vi "Periodic Tasks.vi"   [LabVIEW 2016]
doc: "This VI runs in parallel to other tasks. It can contain as many user-defined periodic loops as you need. These can carry out PID or other sorts of timed response."
uses:
  <vilib>/Rock Robotics/WPI/Solenoid/WPI_SolenoidValue.ctl
  Robot Global Data.vi
  <vilib>/Rock Robotics/WPI/Solenoid/WPI_SolenoidSetEnum.vi
  <vilib>/addons/control/pid/pid.llb/PID (DBL).vi
  <vilib>/addons/control/pid/NI_PID_pid.lvlib
types:
  T1 = typedef "WPI_MotorControlDeviceRef.ctl" = cluster{"DeviceStatus":errorcluster, "Type":T2, "PWM":cluster{"PWM Channel":T3, "DeadBand":T4}, "CAN":cluster{"Device Number":u8, "SetOutput VI Ref":variant, "GetOutput VI Ref":variant, "Enable VI Ref":variant, "Disable VI Ref":variant, "Data":variant}, "Invert":bool}
  T2 = typedef "WPI_MotorControlType.ctl" = enum16{"PWM", "CAN"}
  T3 = typedef "FPGA_DIOPWMChannel.ctl" = enum8{"PWM 0", "PWM 1", "PWM 2", "PWM 3", "PWM 4", "PWM 5", "PWM 6", "PWM 7", "PWM 8", "PWM 9", "PWM MXP 0", "PWM MXP 1", "PWM MXP 2", "PWM MXP 3", "PWM MXP 4", "PWM MXP 5", "PWM MXP 6", "PWM MXP 7", "PWM MXP 8", "PWM MXP 9", "Invalid"}
  T4 = typedef "WPI_PWMDeadband.ctl" = cluster{"Name":string, "maxPositivePwm":i32, "minPositivePwm":i32, "centerPwm":i32, "maxNegativePwm":i32, "minNegativePwm":i32, "angularRange":u16}
  T5 = typedef "WPI_EncoderDevRef.ctl" = cluster{"DevStatus":errorcluster, "EncoderIndex":T6, "CounterIndex":T7, "DistancePerCount":dbl, "Decoding Type":T8}
  T6 = typedef "FPGA_EncoderIdx.ctl" = enum8{"Enc 0", "Enc 1", "Enc 2", "Enc 3", "Enc 4", "Enc 5", "Enc 6", "Enc 7", "Invalid"}
  T7 = typedef "FPGA_CounterCtrSystemIndex.ctl" = enum8{"Ctr 0", "Ctr 1", "Ctr 2", "Ctr 3", "Ctr 4", "Ctr 5", "Ctr 6", "Ctr 7", "Invalid"}
  T8 = typedef "WPI_EncoderType.ctl" = enum16{"1x", "2x", "4x"}
  T9 = typedef "WPI_SolenoidDevRef.ctl" = cluster{"DevStatus":errorcluster, "Pneumatics Control Module":u8, "Forward Solenoid Channel":T10, "Reverse Solenoid Channel":T10}
  T10 = typedef "WPI_SolenoidChannel.ctl" = enum8{"Solenoid 0", "Solenoid 1", "Solenoid 2", "Solenoid 3", "Solenoid 4", "Solenoid 5", "Solenoid 6", "Solenoid 7", "Invalid"}
  T11 = typedef "WPI_PotentiometerDevRef.ctl" = cluster{"DevStatus":errorcluster, "Analog Channel":T12, "Invert Output":bool}
  T12 = typedef "FPGA_AIChannel.ctl" = enum8{"AI 0", "AI 1", "AI 2", "AI 3", "AI MXP 0", "AI MXP 1", "AI MXP 2", "AI MXP 3", "Invalid"}
  T13 = typedef "WPI_SolenoidValue.ctl" = enum16{"Off", "On", "Forward", "Reverse"}
  T14 = cluster{"proportional gain (Kc)":dbl, "integral time (Ti, min)":dbl, "derivative time (Td, min)":dbl}
  T15 = cluster{"Distance (ft)":dbl, "Score":dbl, "Normalized":cluster{"Center":cluster{dbl, dbl}, "Rectangle":cluster{"Numeric":dbl, "Numeric 2":dbl, "Numeric 3":dbl, "Numeric 5":dbl}}, "Pixels":cluster{"Center":cluster{dbl, dbl}, "Rectangle":cluster{"Numeric":dbl, "Numeric 2":dbl, "Numeric 3":dbl, "Numeric 5":dbl}}}
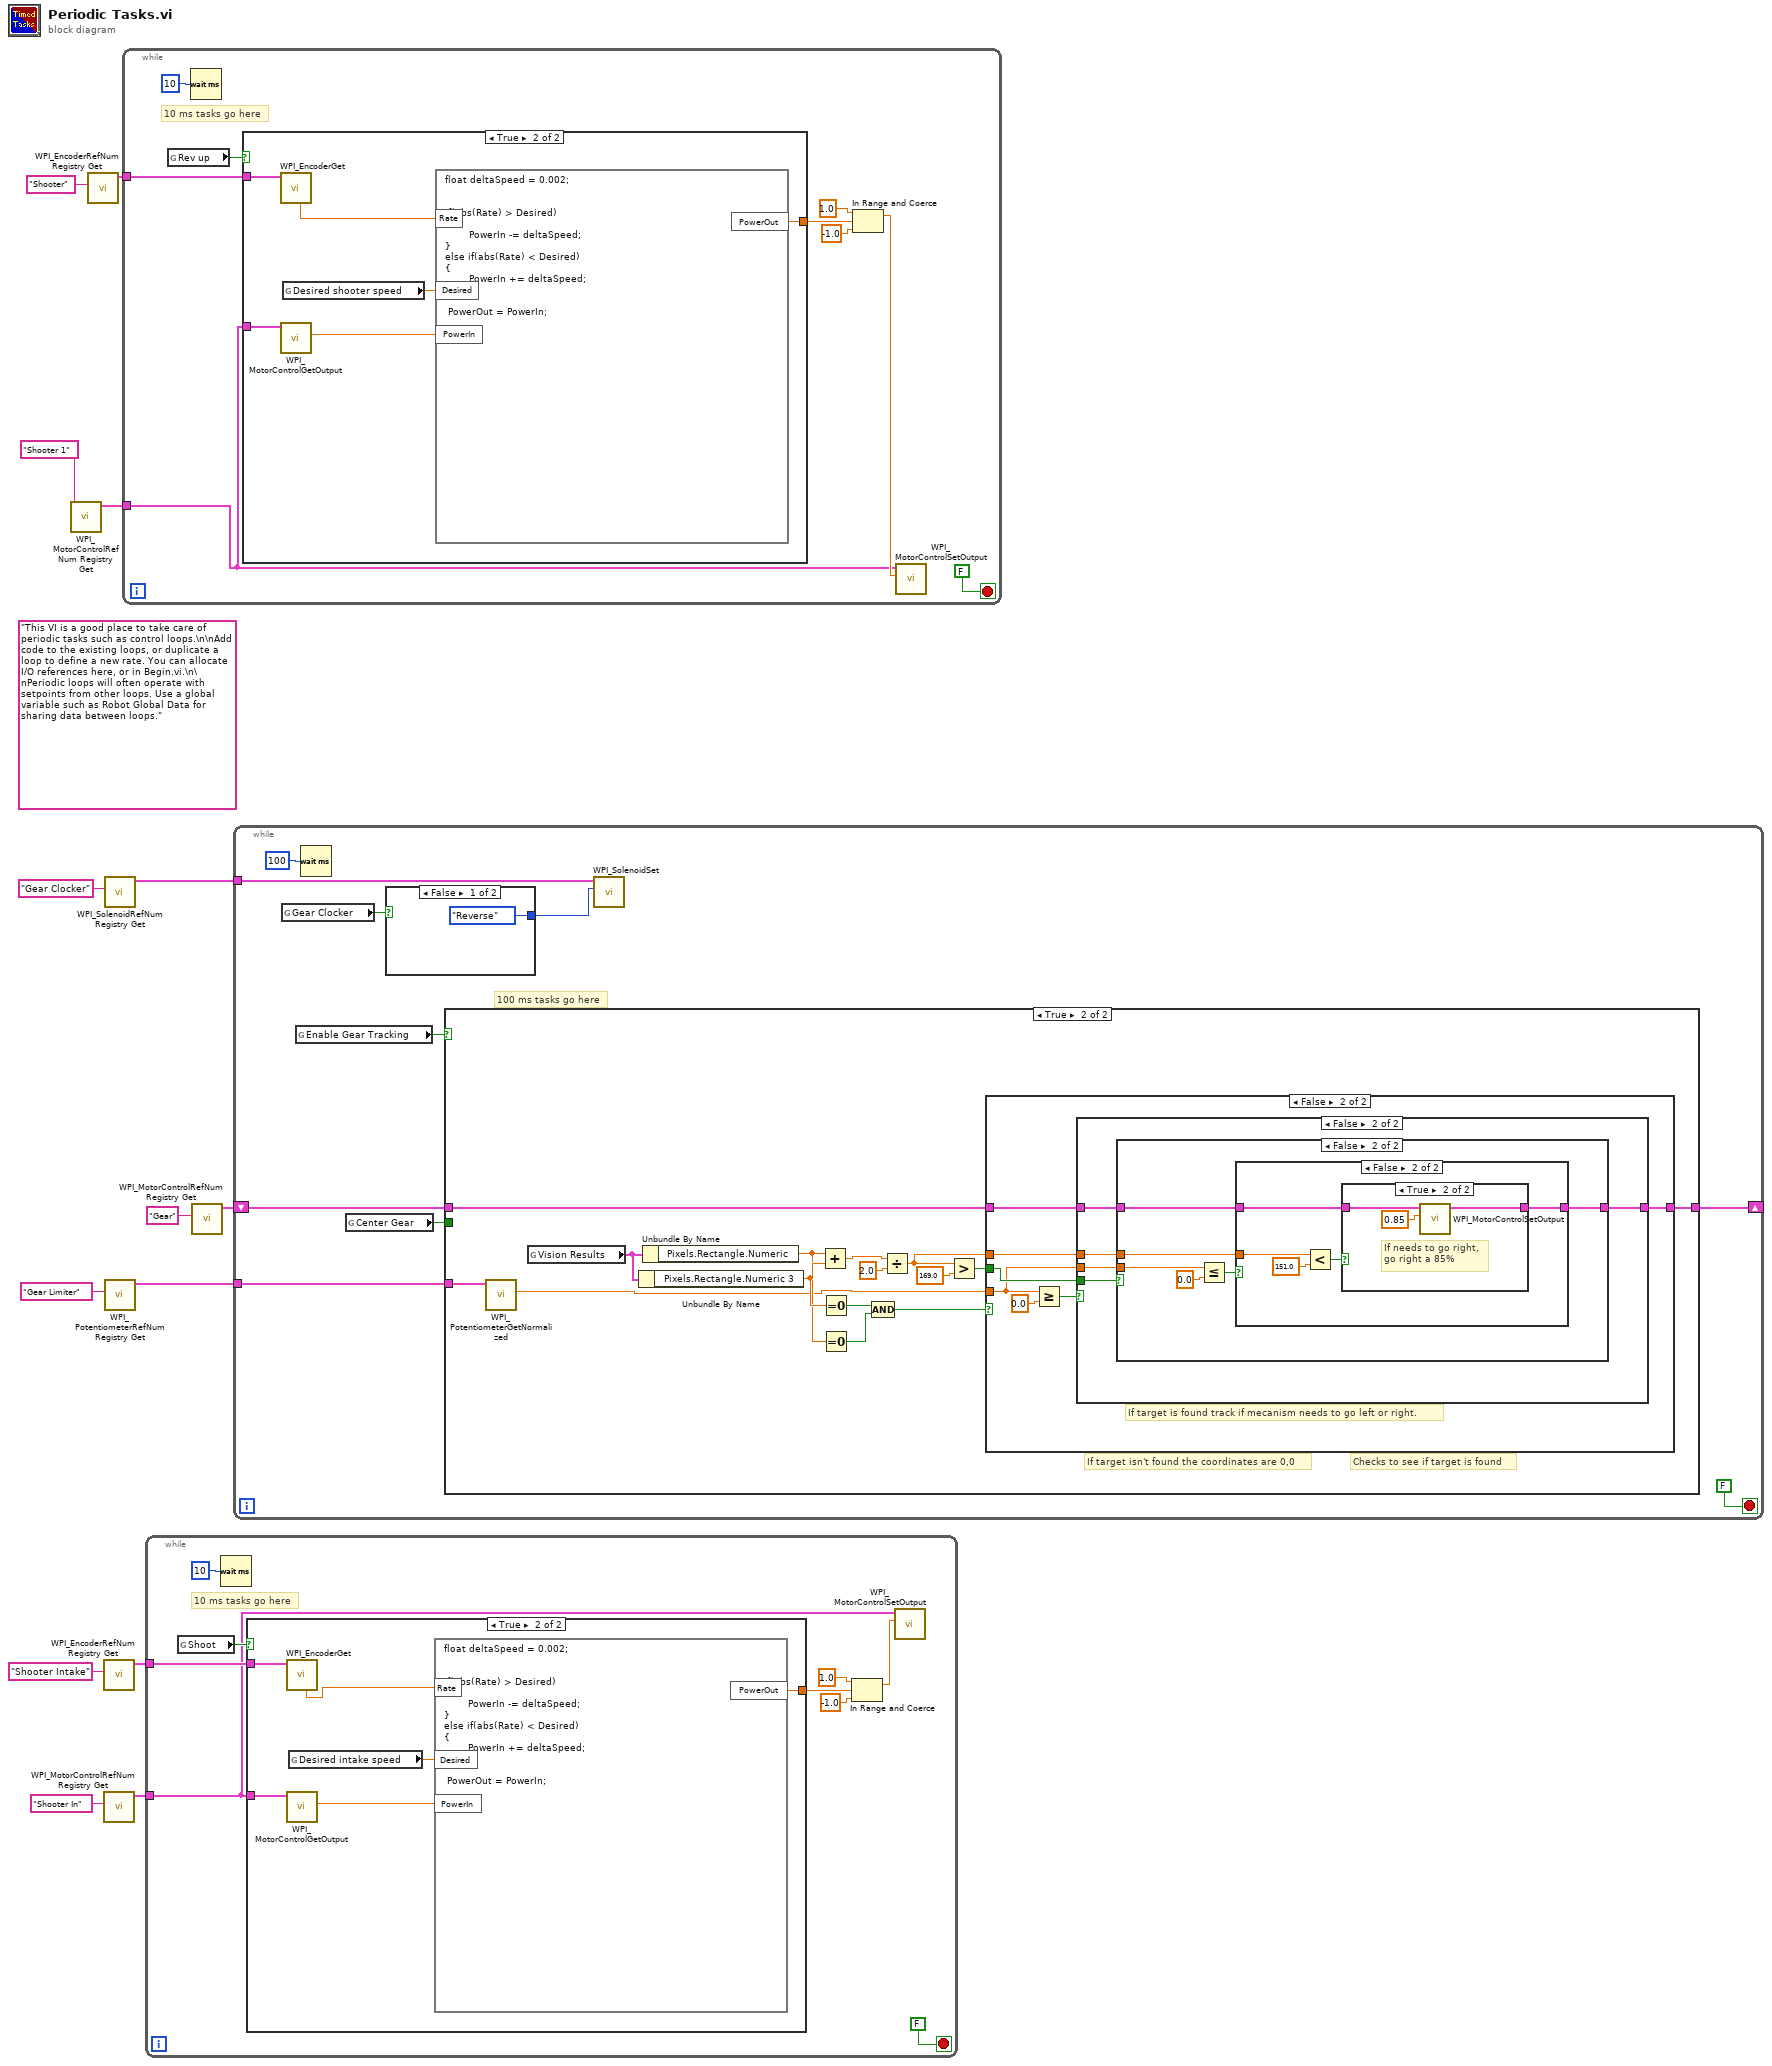
[diagram p0: block diagram]
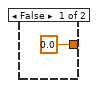
[diagram p2: hidden frame]
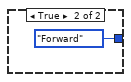
[diagram p3: hidden frame]
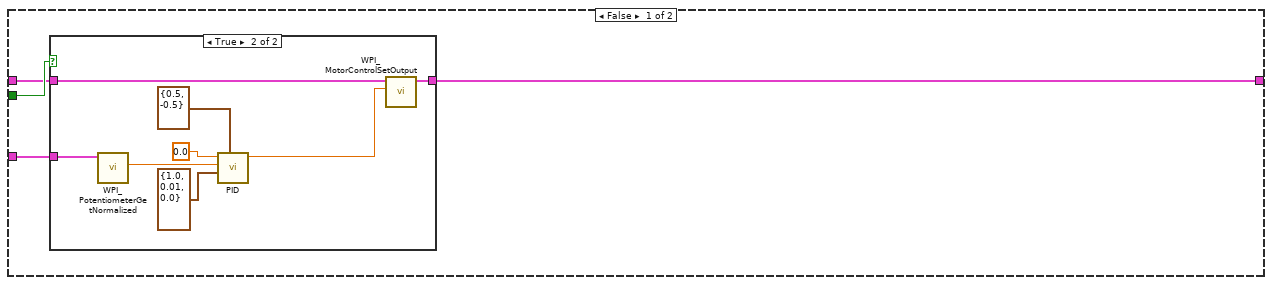
[diagram p4: hidden frame]
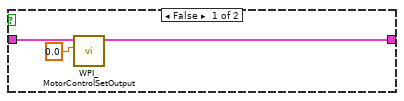
[diagram p5: hidden frame]
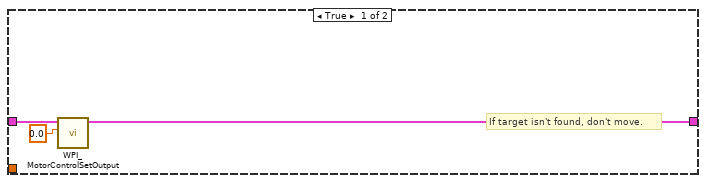
[diagram p6: hidden frame]
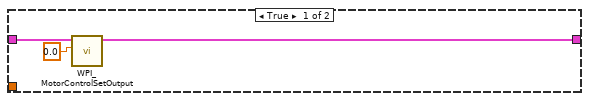
[diagram p7: hidden frame]
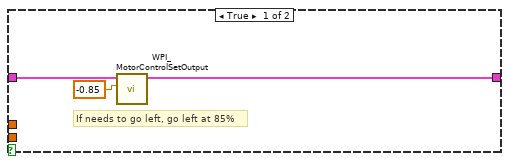
[diagram p8: hidden frame]
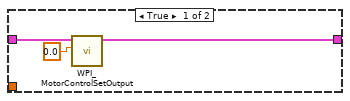
[diagram p9: hidden frame]
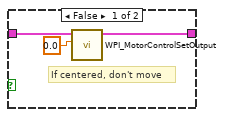
[diagram p10: hidden frame]
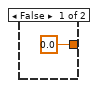
[diagram p11: hidden frame]
diagram:
  (unwired) "This VI is a good place to take care of periodic tasks such as control loops.\n\nAdd code to the existing loops, or duplicate a loop to define a new rate. You can allocate I/O references here, or in Begin.vi.\n\nPeriodic loops will often operate with setpoints from other loops. Use a global variable such as Robot Global Data for sharing data between loops."
  n1 = call <vilib>:"WPI_MotorControlRefNum Registry Get.vi"("refnum name"="Shooter 1") -> ("MotorControlDevRef"=w2:T1)  [unwired: 9 in, 1 out]
  n2 = call <vilib>:"WPI_EncoderRefNum Registry Get.vi"("refnum name"="Shooter") -> ("EncoderDevRef"=w7:T5)  [unwired: 9 in, 1 out]
  n3 = call <vilib>:"WPI_EncoderRefNum Registry Get.vi"("refnum name"="Shooter Intake") -> ("EncoderDevRef"=w6:T5)  [unwired: 9 in, 1 out]
  n4 = call <vilib>:"WPI_MotorControlRefNum Registry Get.vi"("refnum name"="Shooter In") -> ("MotorControlDevRef"=w5:T1)  [unwired: 9 in, 1 out]
  n5 = call <vilib>:"WPI_SolenoidRefNum Registry Get.vi"("refnum name"="Gear Clocker") -> ("SolenoidDevRef"=w9:T9)  [unwired: 9 in, 1 out]
  n6 = call <vilib>:"WPI_PotentiometerRefNum Registry Get.vi"("refnum name"="Gear Limiter") -> ("PotDevRef"=w11:T11)  [unwired: 9 in, 1 out]
  n7 = while {
    tunnel: w7 -> [w21]
    tunnel: w2 -> [w15]
    stop <- FALSE stop-if-true
    # "10 ms tasks go here"
    n8 = global read "Robot Global Data.vi" "Rev up"() -> (w20:bool)
    n9 = Wait (ms)(milliseconds to wait=u32 10) -> ()  [unwired: 1 out]
    n10 = case shown="True" w20 {
      tunnel: w21 -> [_ w30]
      tunnel: w15 -> [_ w26]
      tunnel: [0.0 w25] -> w19
      frame False {
      }
      frame True {
        n11 = call <vilib>:"WPI_EncoderGet.vi"("EncoderDevRef"=w30) -> ("Rate"=w29:dbl)  [unwired: 5 in, 5 out]
        n12 = call <vilib>:"WPI_MotorControlGetOutput.vi"("MotorControlDevRef"=w26) -> ("Output"=w27:dbl)  [unwired: 8 in, 2 out]
        n13 = global read "Robot Global Data.vi" "Desired shooter speed"() -> (w28:dbl)
        n14 = formula code="float deltaSpeed = 0.002;\n\n\nif(abs(Rate) > Desired)\n{\n        PowerIn -= deltaSpeed;\n}\nelse if(abs(Rate) < Desired)\n{\n        PowerIn += deltaSpeed;\n}\n\n PowerOut = PowerIn;"("Rate"=w29, "Desired"=w28, "PowerIn"=w27) -> ("PowerOut"=w25:dbl)
      }
    }
    n15 = In Range and Coerce(upper limit=1.0, x=w19, lower limit=-1.0) -> (coerced(x)=w16:dbl)  [unwired: 1 out]
    n16 = call <vilib>:"WPI_MotorControlSetOutput.vi"("Output"=w16, "MotorControlDevRef"=w15) -> ()  [unwired: 7 in, 3 out]
  }
  n17 = while {
    tunnel: w6 -> [w37]
    tunnel: w5 -> [w35]
    stop <- FALSE stop-if-true
    # "10 ms tasks go here"
    n18 = global read "Robot Global Data.vi" "Shoot"() -> (w36:bool)
    n19 = Wait (ms)(milliseconds to wait=u32 10) -> ()  [unwired: 1 out]
    n20 = case shown="True" w36 {
      tunnel: w37 -> [_ w46]
      tunnel: w35 -> [_ w42]
      tunnel: [0.0 w41] -> w34
      frame False {
      }
      frame True {
        n21 = call <vilib>:"WPI_EncoderGet.vi"("EncoderDevRef"=w46) -> ("Rate"=w45:dbl)  [unwired: 5 in, 5 out]
        n22 = call <vilib>:"WPI_MotorControlGetOutput.vi"("MotorControlDevRef"=w42) -> ("Output"=w43:dbl)  [unwired: 8 in, 2 out]
        n23 = global read "Robot Global Data.vi" "Desired intake speed"() -> (w44:dbl)
        n24 = formula code="float deltaSpeed = 0.002;\n\n\nif(abs(Rate) > Desired)\n{\n        PowerIn -= deltaSpeed;\n}\nelse if(abs(Rate) < Desired)\n{\n        PowerIn += deltaSpeed;\n}\n\n PowerOut = PowerIn;"("Rate"=w45, "Desired"=w44, "PowerIn"=w43) -> ("PowerOut"=w41:dbl)
      }
    }
    n25 = In Range and Coerce(upper limit=1.0, x=w34, lower limit=-1.0) -> (coerced(x)=w33:dbl)  [unwired: 1 out]
    n26 = call <vilib>:"WPI_MotorControlSetOutput.vi"("Output"=w33, "MotorControlDevRef"=w35) -> ()  [unwired: 7 in, 3 out]
  }
  n27 = call <vilib>:"WPI_MotorControlRefNum Registry Get.vi"("refnum name"="Gear") -> ("MotorControlDevRef"=w13:T1)  [unwired: 9 in, 1 out]
  n28 = while {
    shift-right: [w52] -> _
    shift-left: w13 -> [w54]
    tunnel: w11 -> [w50]
    tunnel: w9 -> [w47]
    stop <- FALSE stop-if-true
    # "100 ms tasks go here"
    n29 = global read "Robot Global Data.vi" "Gear Clocker"() -> (w49:bool)
    n30 = global read "Robot Global Data.vi" "Enable Gear Tracking"() -> (w53:bool)
    n31 = Wait (ms)(milliseconds to wait=u32 100) -> ()  [unwired: 1 out]
    n32 = global read "Robot Global Data.vi" "Center Gear"() -> (w51:bool)
    n33 = case shown="False" w49 {
      tunnel: [WPI_SolenoidValue."Reverse" ("Value") WPI_SolenoidValue."Forward" ("Value")] -> w48
      frame False {
      }
      frame True {
      }
    }
    n34 = case shown="True" w53 {
      tunnel: w54 -> [w60 w82]
      tunnel: [w59 w81] -> w52
      tunnel: w51 -> [w62 _]
      tunnel: w50 -> [w61 w75]
      frame False {
        n35 = case shown="True" w62 {
          tunnel: w61 -> [_ w72]
          tunnel: w60 -> [w64 w67]
          tunnel: [w63 w66] -> w59
          frame False {
            n36 = call <vilib>:"WPI_MotorControlSetOutput.vi"("Output"=0.0, "MotorControlDevRef"=w64) -> ("MotorControlDevRef"=w63:T1)  [unwired: 7 in, 2 out]
          }
          frame True {
            n37 = call <vilib>:"WPI_PotentiometerGetNormalized.vi"("PotDevRef"=w72) -> ("Normalized Value"=w73:dbl)  [unwired: 8 in, 2 out]
            n38 = call-poly <vilib>:"PID.vi"("output range"=cluster{"output high":dbl, "output low":dbl} {"output high"=0.5, "output low"=-0.5}, "PID gains"=T14 {"proportional gain (Kc)"=1.0, "integral time (Ti, min)"=0.01, "derivative time (Td, min)"=0.0}, "process variable"=w73, "setpoint"=0.0) -> ("output"=w68:dbl)  [unwired: 6 in, 1 out]
            n39 = call <vilib>:"WPI_MotorControlSetOutput.vi"("Output"=w68, "MotorControlDevRef"=w67) -> ("MotorControlDevRef"=w66:T1)  [unwired: 7 in, 2 out]
          }
        }
      }
      frame True {
        # "If target isn't found the coordinates are 0,0"
        # "Checks to see if target is found"
        n40 = call <vilib>:"WPI_PotentiometerGetNormalized.vi"("PotDevRef"=w75) -> ("Normalized Value"=w74:dbl)  [unwired: 8 in, 2 out]
        n41 = global read "Robot Global Data.vi" "Vision Results"() -> (w83:T15)
        n42 = Unbundle By Name(w83) -> ("Pixels.Rectangle.Numeric 3"=w80:dbl)
        n43 = Unbundle By Name(w83) -> ("Pixels.Rectangle.Numeric"=w79:dbl)
        n44 = Add(x=w79, y=w80) -> (x+y=w87:dbl)
        n45 = Equal To 0?(x=w80) -> (x = 0?=w77:bool)
        n46 = Equal To 0?(x=w79) -> (x = 0?=w78:bool)
        n47 = Compound Arithmetic op=AND(w77, w78) -> (w76:bool)
        n48 = Divide(x=w87, y=2.0) -> (x/y=w85:dbl)
        n49 = Greater?(x=w85, y=169.0) -> (0:w84:bool)
        n50 = case shown="False" w76 {
          tunnel: w85 -> [_ w98]
          tunnel: w84 -> [_ w97]
          tunnel: w82 -> [w91 w96]
          tunnel: [w89 w95] -> w81
          tunnel: w74 -> [_ w94]
          frame True {
            # "If target isn't found, don't move."
            n51 = call <vilib>:"WPI_MotorControlSetOutput.vi"("Output"=0.0, "MotorControlDevRef"=w91) -> ("MotorControlDevRef"=w89:T1)  [unwired: 7 in, 2 out]
          }
          frame False {
            # "If target is found track if mecanism needs to go left or right."
            n52 = Greater Or Equal?(x=w94, y=0.0) -> (x >= y?=w92:bool)
            n53 = case shown="False" w92 {
              tunnel: w98 -> [_ w106]
              tunnel: w97 -> [_ w105]
              tunnel: w96 -> [w101 w104]
              tunnel: [w100 w103] -> w95
              tunnel: w94 -> [_ w102]
              frame True {
                n54 = call <vilib>:"WPI_MotorControlSetOutput.vi"("Output"=0.0, "MotorControlDevRef"=w101) -> ("MotorControlDevRef"=w100:T1)  [unwired: 7 in, 2 out]
              }
              frame False {
                n55 = case shown="False" w105 {
                  tunnel: w106 -> [_ w115]
                  tunnel: w104 -> [w109 w114]
                  tunnel: [w107 w113] -> w103
                  tunnel: w102 -> [_ w110]
                  frame True {
                    # "If needs to go left, go left at 85%"
                    n56 = call <vilib>:"WPI_MotorControlSetOutput.vi"("Output"=-0.85, "MotorControlDevRef"=w109) -> ("MotorControlDevRef"=w107:T1)  [unwired: 7 in, 2 out]
                  }
                  frame False {
                    n57 = Less Or Equal?(x=w110, y=0.0) -> (x <= y?=w112:bool)
                    n58 = case shown="False" w112 {
                      tunnel: w115 -> [_ w121]
                      tunnel: w114 -> [w117 w120]
                      tunnel: [w116 w119] -> w113
                      frame True {
                        n59 = call <vilib>:"WPI_MotorControlSetOutput.vi"("Output"=0.0, "MotorControlDevRef"=w117) -> ("MotorControlDevRef"=w116:T1)  [unwired: 7 in, 2 out]
                      }
                      frame False {
                        n60 = Less?(x=w121, y=151.0) -> (x < y?=w122:bool)
                        n61 = case shown="True" w122 {
                          tunnel: w120 -> [w125 w129]
                          tunnel: [w124 w127] -> w119
                          frame False {
                            # "If centered, don't move"
                            n62 = call <vilib>:"WPI_MotorControlSetOutput.vi"("Output"=0.0 ("Left axis value"), "MotorControlDevRef"=w125) -> ("MotorControlDevRef"=w124:T1)  [unwired: 7 in, 2 out]
                          }
                          frame True {
                            # "If needs to go right,\ngo right a 85%"
                            n63 = call <vilib>:"WPI_MotorControlSetOutput.vi"("Output"=0.85, "MotorControlDevRef"=w129) -> ("MotorControlDevRef"=w127:T1)  [unwired: 7 in, 2 out]
                          }
                        }
                      }
                    }
                  }
                }
              }
            }
          }
        }
      }
    }
    n64 = call-poly <vilib>:"WPI_SolenoidSet.vi"("Value"=w48, "SolenoidDevRef"=w47) -> ()  [unwired: 8 in, 2 out]
  }
